vi "Resize and Align.vi"(9 "number of channels":i32, 10 "Refnums for Resizing and Alignment":T4, 11 "State in":T1={"Graph Visible Items"={"Plot Legend"=FALSE, "Scale Legend"=FALSE, "Graph Palette"=FALSE, "Cursor Legend"=FALSE, "X Scrollbar"=FALSE}, "View Table"=FALSE, "Table Visible Items"={"Vertical Scrollbar"=FALSE, "Horizontal Scrollbar"=FALSE, "Row Headers"=FALSE, "Column Headers"=FALSE, "Vertical Lines"=FALSE, "Horizontal Lines"=FALSE}, "Header Font"={"Font Name"="", "Size"=0, "Bold"=FALSE, "Italic"=FALSE, "Underline"=FALSE, "Strikeout"=FALSE, "Color"=0}, "Cell Font"={"Font Name"="", "Size"=0, "Bold"=FALSE, "Italic"=FALSE, "Underline"=FALSE, "Strikeout"=FALSE, "Color"=0}, "Description and Tip..."={"Description"="", "Tip"=""}, "Moveable Splitter Position"=0, "Measurement Cursor Configuration"={"XY"={"enable XY"=FALSE, "Position (X)"=[], "Type"=enum."Absolute", "Y reference"=0.0, "color"=0}, "band"={"enable band"=FALSE, "B1"=0.0, "B2"=0.0, "Fixed bandwidth (B2-B1)"=0.0, "B1 color"=0, "B2 color"=0}, "harmonic"={"enable harmonics"=FALSE, "X reference (1X)"=0.0, "Maximum"=0, "Subset"=enum."All", "1X color"=0, "MX color"=0}, "sideband"={"enable sideband"=FALSE, "X center (C)"=0.0, "Sidebands"=0, "X spacing (s)"=0.0, "Center color"=0, "Sideband color"=0}}, "Cursors"={"List"=[], "Tags"=[]}, "X Increment"=0.0, "X Scale"={"Label Visible"=FALSE, "Label Text"="", "Mapping Mode"=0, "Format String"=""}, "Y Scale"={"Label Visible"=FALSE, "Label Text"="", "Mapping Mode"=0, "Format String"=""}, "Colors"={"background"=16777215, "major grid"=8355711, "minor grid"=12632256, "font"=0}, "desired spectrum view"={"scaling"={"linear/dB"=enum."no change", "dB reference"=0.0, "power/magnitude"=enum."no change", "view"=enum."no change"}, "spectral density"=enum."no change"}, "Plot Color Wheel"=[3381759, 32768, 982784, 4375295, 13827953, 13457919, 16757522, 4343295, 16728758, 12095254], "Plots"=[], "registered user events"=variant, "Lock 1X to Peak"=FALSE} caption="State" {"Y Scale"."Mapping Mode" items=["Linear", "Logarithmic", "dB"]; "X Scale"."Mapping Mode" items=["Linear", "Logarithmic"]}) -> (0 "error out":errorcluster, 3 "State out":T1={"Graph Visible Items"={"Plot Legend"=FALSE, "Scale Legend"=FALSE, "Graph Palette"=FALSE, "Cursor Legend"=FALSE, "X Scrollbar"=FALSE}, "View Table"=FALSE, "Table Visible Items"={"Vertical Scrollbar"=FALSE, "Horizontal Scrollbar"=FALSE, "Row Headers"=FALSE, "Column Headers"=FALSE, "Vertical Lines"=FALSE, "Horizontal Lines"=FALSE}, "Header Font"={"Font Name"="", "Size"=0, "Bold"=FALSE, "Italic"=FALSE, "Underline"=FALSE, "Strikeout"=FALSE, "Color"=0}, "Cell Font"={"Font Name"="", "Size"=0, "Bold"=FALSE, "Italic"=FALSE, "Underline"=FALSE, "Strikeout"=FALSE, "Color"=0}, "Description and Tip..."={"Description"="", "Tip"=""}, "Moveable Splitter Position"=0, "Measurement Cursor Configuration"={"XY"={"enable XY"=FALSE, "Position (X)"=[], "Type"=enum."Absolute", "Y reference"=0.0, "color"=0}, "band"={"enable band"=FALSE, "B1"=0.0, "B2"=0.0, "Fixed bandwidth (B2-B1)"=0.0, "B1 color"=0, "B2 color"=0}, "harmonic"={"enable harmonics"=FALSE, "X reference (1X)"=0.0, "Maximum"=0, "Subset"=enum."All", "1X color"=0, "MX color"=0}, "sideband"={"enable sideband"=FALSE, "X center (C)"=0.0, "Sidebands"=0, "X spacing (s)"=0.0, "Center color"=0, "Sideband color"=0}}, "Cursors"={"List"=[], "Tags"=[]}, "X Increment"=0.0, "X Scale"={"Label Visible"=FALSE, "Label Text"="", "Mapping Mode"=0, "Format String"=""}, "Y Scale"={"Label Visible"=FALSE, "Label Text"="", "Mapping Mode"=0, "Format String"=""}, "Colors"={"background"=16777215, "major grid"=8355711, "minor grid"=12632256, "font"=0}, "desired spectrum view"={"scaling"={"linear/dB"=enum."no change", "dB reference"=0.0, "power/magnitude"=enum."no change", "view"=enum."no change"}, "spectral density"=enum."no change"}, "Plot Color Wheel"=[3381759, 32768, 982784, 4375295, 13827953, 13457919, 16757522, 4343295, 16728758, 12095254], "Plots"=[], "registered user events"=variant, "Lock 1X to Peak"=FALSE} caption="State" {"Y Scale"."Mapping Mode" items=["Linear", "Logarithmic", "dB"]; "X Scale"."Mapping Mode" items=["Linear", "Logarithmic"]})   [LabVIEW 2017, in "Octave with Cursors.xctl"]
doc: "Based on moveable splitter position and pane sizes, resize the graph and table and align table with plot area."
uses:
  <vilib>/addons/_XControls/Octave with Cursors/Octave with Cursors.xctl
  <vilib>/addons/_XControls/Octave with Cursors/Controls/Refnums Typedef.ctl
  <vilib>/addons/Sound and Vibration/svt_Controls/subVIs/Multiplot Octave Graph.ctl
  <vilib>/addons/_XControls/Octave with Cursors/Controls/State.ctl
  <vilib>/Utility/miscctls.llb/LVFontTypeDef.ctl
  <vilib>/addons/_XControls/Octave with Cursors/Controls/Measurement Cursor Configuration.ctl
  <vilib>/Utility/miscctls.llb/LVPositionTypeDef.ctl
  <vilib>/Utility/miscctls.llb/LVRowAndColumnTypeDef.ctl
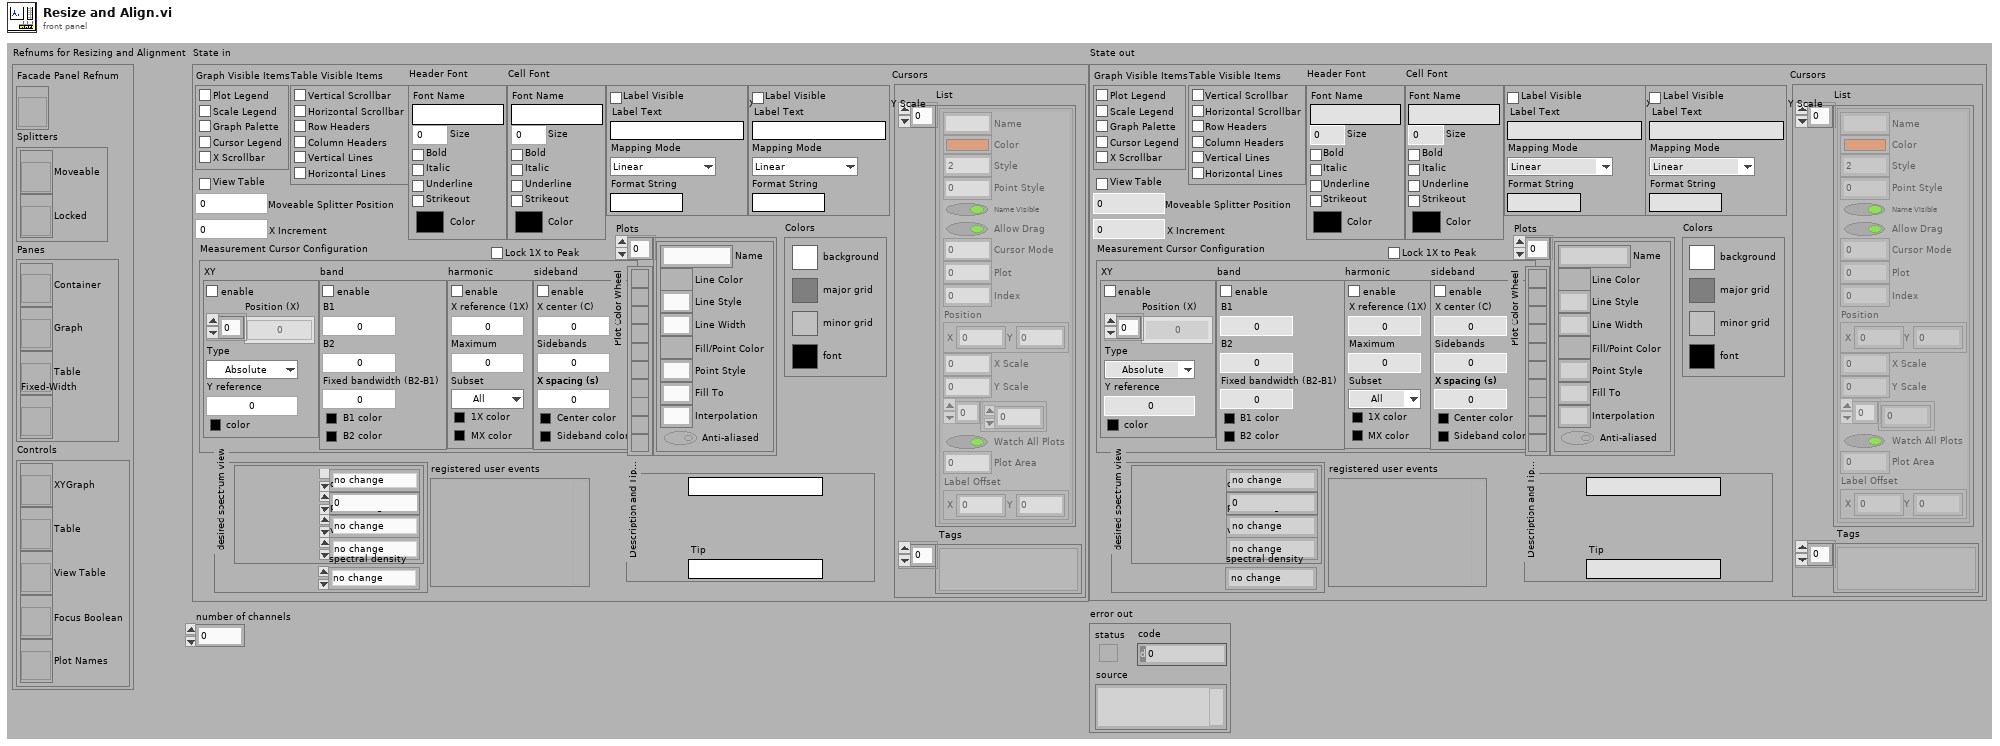
[diagram p1: front panel]
types:
  T1 = typedef "Octave with Cursors.xctl/State.ctl" = cluster{"Graph Visible Items":cluster{"Plot Legend":bool, "Scale Legend":bool, "Graph Palette":bool, "Cursor Legend":bool, "X Scrollbar":bool}, "View Table":bool, "Table Visible Items":cluster{"Vertical Scrollbar":bool, "Horizontal Scrollbar":bool, "Row Headers":bool, "Column Headers":bool, "Vertical Lines":bool, "Horizontal Lines":bool}, "Header Font":T2, "Cell Font":T2, "Description and Tip...":cluster{"Description":string, "Tip":string}, "Moveable Splitter Position":i32, "Measurement Cursor Configuration":T3, "Cursors":cluster{"List":cluster{"Name":string, "Color":u32, "Style":i32, "Point Style":u8, "Name Visible":bool, "Allow Drag":bool, "Cursor Mode":u32, "Plot":i32, "Index":i32, "Position":cluster{"X":dbl, "Y":dbl}, "X Scale":u32, "Y Scale":u32, "Watch Plots":i32[], "Watch All Plots":bool, "Plot Area":i32, "Label Offset":cluster{"X":dbl, "Y":dbl}}[], "Tags":variant[]}, "X Increment":dbl, "X Scale":cluster{"Label Visible":bool, "Label Text":string, "Mapping Mode":u8, "Format String":string}, "Y Scale":cluster{"Label Visible":bool, "Label Text":string, "Mapping Mode":u8, "Format String":string}, "Colors":cluster{"background":u32, "major grid":u32, "minor grid":u32, "font":u32}, "desired spectrum view":cluster{"scaling":cluster{"linear/dB":enum16{"no change", "linear", "dB"}, "dB reference":dbl, "power/magnitude":enum16{"no change", "power", "magnitude"}, "view":enum16{"no change", "rms", "peak", "peak-peak"}}, "spectral density":enum16{"no change", "spectrum", "spectral density"}}, "Plot Color Wheel":u32[], "Plots":cluster{"Name":string, "Line Color":u32, "Line Style":u8, "Line Width":u8, "Fill/Point Color":u32, "Point Style":u8, "Fill To":i16, "Interpolation":u8, "Anti-aliased":bool}[], "registered user events":variant, "Lock 1X to Peak":bool}
  T2 = typedef "LVFontTypeDef.ctl" = cluster{"Font Name":string, "Size":u16, "Bold":bool, "Italic":bool, "Underline":bool, "Strikeout":bool, "Color":u32}
  T3 = typedef "Octave with Cursors.xctl/Measurement Cursor Configuration.ctl" = cluster{"XY":cluster{"enable XY":bool, "Position (X)":dbl[], "Type":enum16{"Absolute", "Relative"}, "Y reference":dbl, "color":u32}, "band":cluster{"enable band":bool, "B1":dbl, "B2":dbl, "Fixed bandwidth (B2-B1)":dbl, "B1 color":u32, "B2 color":u32}, "harmonic":cluster{"enable harmonics":bool, "X reference (1X)":dbl, "Maximum":i32, "Subset":enum16{"All", "Even", "Odd"}, "1X color":u32, "MX color":u32}, "sideband":cluster{"enable sideband":bool, "X center (C)":dbl, "Sidebands":i32, "X spacing (s)":dbl, "Center color":u32, "Sideband color":u32}}
  T4 = typedef "Octave with Cursors.xctl/Refnums Typedef.ctl" = cluster{"Facade Panel Refnum":refnum<vi>, "Splitters":cluster{"Moveable":refnum<vi>, "Locked":refnum<vi>}, "Panes":cluster{"Container":refnum<vi>, "Graph":refnum<vi>, "Table":refnum<vi>, "Fixed-Width":refnum<vi>}, "Controls":cluster{"XYGraph":refnum<vi>, "Table":refnum<vi>, "View Table":refnum<vi>, "Focus Boolean":refnum<vi>, "Plot Names":refnum<vi>}}
  T5 = typedef "LVPositionTypeDef.ctl" = cluster{"Left":i32, "Top":i32}
  T6 = typedef "LVRectTypeDef.ctl" = cluster{"Left":i16, "Top":i16, "Right":i16, "Bottom":i16}
  T7 = typedef "Multiplot Octave Graph.ctl" = cluster{"nominal frequencies [Hz]":dbl[], "band power [dB EU]":dbl[]}[]
  T8 = typedef "LVRowAndColumnTypeDef.ctl" = cluster{"Row":i32, "Column":i32}
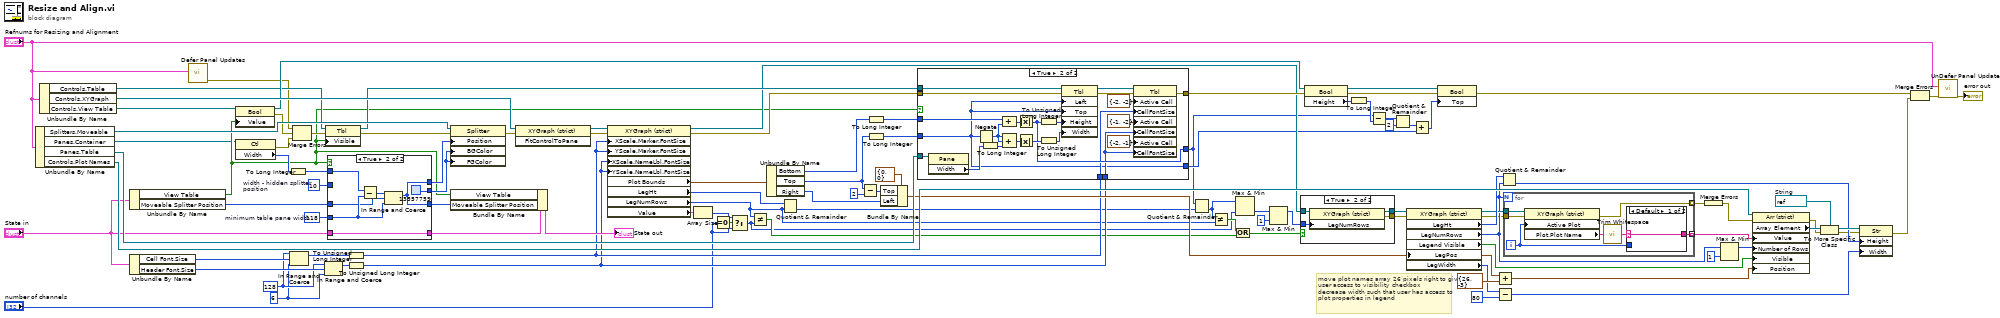
[diagram p0: block diagram]
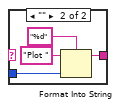
[diagram p3: hidden frame]
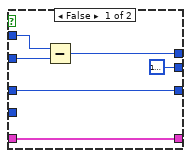
[diagram p4: hidden frame]
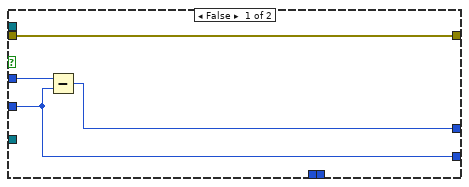
[diagram p5: hidden frame]
diagram:
  w57 = u16 128 ("upper limit")
  w56 = u16 6 ("lower limit")
  w76 = refnum<vi> refnum  # String
  w77 = 118  # minimum table pane width
  w7 = 10  # width - hidden splitter position
  # "move plot names array 26 pixels right to give user access to visibility checkbox\ndecrease width such that user has access to plot properties in legend"
  n1 = Unbundle By Name("Refnums for Resizing and Alignment") -> ("Splitters.Moveable"=w97:refnum<vi>, "Panes.Container"=w5:refnum<vi>, "Panes.Table"=w93:refnum<vi>, "Controls.Plot Names"=w62:refnum<vi>)
  n2 = Unbundle By Name("Refnums for Resizing and Alignment") -> ("Controls.Table"=w17:refnum<vi>, "Controls.XYGraph"=w99:refnum<vi>, "Controls.View Table"=w18:refnum<vi>)
  n3 = Unbundle By Name("State in") -> ("View Table"=w6:bool, "Moveable Splitter Position"=w91:i32)
  n4 = Unbundle By Name("State in") -> ("Cell Font.Size"=w58:u16, "Header Font.Size"=w59:u16)
  n5 = call <vilib>:"Defer Panel Updates.vi"("Refnums for FP Objects"="Refnums for Resizing and Alignment") -> ("error out"=w3:errorcluster)  [unwired: 9 in, 1 out]
  n6 = property class="Bool"(reference=w18, "Value"=w6) -> (reference out=w90:refnum<vi>, error out=w8:errorcluster)  [unwired: 1 in]
  n7 = property class="Ctl"(reference=w5) -> (error out=w98:errorcluster, "Width"=w96:u32)  [unwired: 1 in, 1 out]
  n8 = To Long Integer(number=w96) -> (32bit integer=w79:i32)
  n9 = In Range and Coerce(upper limit=w57, x=w58, lower limit=w56) -> (coerced(x)=w53:u16)  [unwired: 1 out]
  n10 = Merge Errors(w3, w8, w98) -> (w11:errorcluster)
  n11 = In Range and Coerce(upper limit=w57, x=w59, lower limit=w56) -> (coerced(x)=w52:u16)  [unwired: 1 out]
  n12 = property class="Tbl"(reference=w17, error in=w11, "Visible"=w6) -> (reference out=w54:refnum<vi>, error out=w55:errorcluster)
  n13 = case shown="True" w6 {
    tunnel: w79 -> [w106 w114]
    tunnel: [w104 w115] -> w95
    tunnel: [u32 16777216 ("Color Box") u32 13557759 ("Color Box")] -> w94
    tunnel: [w108 w115] -> w78
    tunnel: w91 -> [w108 w110]
    tunnel: w77 -> [_ w113]
    tunnel: "State in" -> [w107 w112]
    tunnel: [w107 w112] -> w10
    tunnel: w7 -> [w105 _]
    frame False {
      n14 = Subtract(x=w106, y=w105) -> (x-y=w104:i32)
    }
    frame True {
      n15 = Subtract(x=w114, y=w113) -> (x-y=w116:i32)
      n16 = In Range and Coerce(upper limit=w116, x=w110, lower limit=w113) -> (coerced(x)=w115:i32)  [unwired: 1 out]
    }
  }
  n17 = To Unsigned Long Integer(number=w53) -> (unsigned 32bit integer=w51:u32)
  n18 = To Unsigned Long Integer(number=w52) -> (unsigned 32bit integer=w50:u32)
  n19 = property class="Splitter"(reference=w97, error in=w55, "Position"=w95, "BGColor"=w94, "FGColor"=w94) -> (error out=w101:errorcluster)  [unwired: 1 out]
  n20 = Bundle By Name(cluster=w10, "View Table"=w6, "Moveable Splitter Position"=w78) -> (→"State out":T1)
  n21 = invoke class="XYGraph (strict)" method="FitControlToPane"(reference=w99, error in=w101) -> (reference out=w103:refnum<vi>, error out=w102:errorcluster)  [unwired: 1 in, 1 out]
  n22 = property class="XYGraph (strict)"(reference=w103, error in=w102, "XScale.Marker.FontSize"=w51, "YScale.Marker.FontSize"=w51, "XScale.NameLbl.FontSize"=w50, "YScale.NameLbl.FontSize"=w50) -> (reference out=w38:refnum<vi>, error out=w100:errorcluster, "Plot Bounds"=w46:T6, "LegHt"=w24:u32, "LegNumRows"=w20:u32, "Value"=w28:T7)
  n23 = Array Size(array=w28) -> (size(s)=w26:i32)
  n24 = Equal To 0?(x="number of channels") -> (x = 0?=w27:bool)
  n25 = Select(t=w26, s=w27, f="number of channels") -> (s? t:f=w13:i32)
  n26 = Not Equal?(x=w20, y=w13) -> (x != y?=w29:bool)
  n27 = Unbundle By Name(w46) -> ("Bottom"=w45:i16, "Top"=w68:i16, "Right"=w69:i16)
  n28 = Quotient & Remainder(x=w24, y=w20) -> (floor(x/y)=w22:u32)  [unwired: 1 out]
  n29 = Subtract(x=w68, y=i16 2) -> (x-y=w67:i16)
  n30 = To Long Integer(number=w45) -> (32bit integer=w80:i32)
  n31 = To Long Integer(number=w68) -> (32bit integer=w49:i32)
  n32 = Bundle By Name(cluster=T5 {"Left"=0, "Top"=0} ("Legend:Position"), "Top"=w67, "Left"=w69) -> (w60:T5)
  n33 = case shown="True" w6 {
    tunnel: w54 -> [_ w142]
    tunnel: w49 -> [w117 w121]
    tunnel: w80 -> [w119 w141]
    tunnel: w93 -> [_ w139]
    tunnel: w100 -> [w120 w136]
    tunnel: [w120 w122] -> w87
    tunnel: [w118 w128] -> w21
    tunnel: w51 -> [_ w126]
    tunnel: w50 -> [_ w123]
    tunnel: [w117 w121] -> w23
    frame False {
      n34 = Subtract(x=w119, y=w117) -> (x-y=w118:i32)
    }
    frame True {
      n35 = property class="Pane"(reference=w139) -> ("Width"=w138:u32)  [unwired: 1 in, 2 out]
      n36 = Negate(x=w121) -> (-x=w133:i32)
      n37 = To Long Integer(number=w138) -> (32bit integer=w134:i32)
      n38 = Compound Arithmetic op=ADD(w141, w133) -> (w140:i32)
      n39 = Compound Arithmetic op=ADD(w133, w133, w134) -> (w137:i32)
      n40 = Absolute Value(x=w140) -> (abs(x)=w128:i32)
      n41 = Absolute Value(x=w137) -> (abs(x)=w131:i32)
      n42 = To Unsigned Long Integer(number=w128) -> (unsigned 32bit integer=w135:u32)
      n43 = To Unsigned Long Integer(number=w131) -> (unsigned 32bit integer=w132:u32)
      n44 = property class="Tbl"(reference=w142, error in=w136, "Left"=w121, "Top"=w121, "Height"=w135, "Width"=w132) -> (reference out=w130:refnum<vi>, error out=w129:errorcluster)
      n45 = property class="Tbl"(reference=w130, error in=w129, "Active Cell"=T8 {"Row"=-2, "Column"=-2} ("Active Cell:Active Cell"), "CellFontSize"=w126, "Active Cell"=T8 {"Row"=-1, "Column"=-2} ("Active Cell:Active Cell"), "CellFontSize"=w123, "Active Cell"=T8 {"Row"=-2, "Column"=-1} ("Active Cell:Active Cell"), "CellFontSize"=w123) -> (error out=w122:errorcluster)  [unwired: 1 out]
    }
  }
  n46 = Quotient & Remainder(x=w21, y=w22) -> (floor(x/y)=w14:u32)  [unwired: 1 out]
  n47 = Not Equal?(x=w14, y=w20) -> (x != y?=w19:bool)
  n48 = Or(x=w19, y=w29) -> (x .or. y?=w30:bool)
  n49 = Max & Min(x=w14, y=w13) -> (min(x,y)=w15:u32)  [unwired: 1 out]
  n50 = Max & Min(x=w15, y=u32 1 ("lower limit")) -> (max(x,y)=w12:u32)  [unwired: 1 out]
  n51 = case shown="True" w30 {
    tunnel: w38 -> [w143 w147]
    tunnel: [w143 w146] -> w37
    tunnel: w12 -> [_ w145]
    tunnel: [_ w144] -> w36
    frame False {
    }
    frame True {
      n52 = property on="Property Node" class="XYGraph (strict)"(reference=w147, "LegNumRows"=w145) -> (reference out=w146:refnum<vi>, error out=w144:errorcluster)  [unwired: 1 in]
    }
  }
  n53 = property class="Bool"(reference=w90, error in=w87) -> (reference out=w89:refnum<vi>, error out=w86:errorcluster, "Height"=w88:u32)
  n54 = To Long Integer(number=w88) -> (32bit integer=w85:i32)
  n55 = Subtract(x=w21, y=w85) -> (x-y=w84:i32)
  n56 = Quotient & Remainder(x=w84, y=2) -> (floor(x/y)=w82:i32)  [unwired: 1 out]
  n57 = property on="Property Node" class="XYGraph (strict)"(reference=w37, error in=w36, "LegPos"=w60) -> (reference out=w43:refnum<vi>, error out=w35:errorcluster, "LegHt"=w47:u32, "LegNumRows"=w39:u32, "Legend Visible"=w48:bool, "LegWidth"=w61:u32)
  n58 = Add(x=w82, y=w23) -> (x+y=w81:i32)
  n59 = property class="Bool"(reference=w89, error in=w86, "Top"=w81) -> (error out=w41:errorcluster)  [unwired: 1 out]
  n60 = Add(x=w60, y=T5 {"Left"=26, "Top"=-3}) -> (x+y=w72:T5)
  n61 = Subtract(x=w61, y=u32 80) -> (x-y=w63:u32)
  n62 = Quotient & Remainder(x=w47, y=w39) -> (floor(x/y)=w66:u32)  [unwired: 1 out]
  n63 = for {
    N: w39 -> [_]
    tunnel: [w154] -> w64 mode=indexing
    tunnel: w43 -> [w153]
    tunnel: w35 -> [w149]
    tunnel: [w148] -> w34 mode=indexing
    i -> [w150]
    n64 = property on="Property Node" class="XYGraph (strict)"(reference=w153, error in=w149, "Active Plot"=w150) -> (error out=w148:errorcluster, "Plot.Plot Name"=w152:string)  [unwired: 1 out]
    n65 = call <vilib>:"Trim Whitespace.vi"("string"=w152) -> ("trimmed string"=w151:string)  [unwired: 1 in]
    n66 = case shown="Default" w151 {
      selector: w151 -> [w155 _]
      tunnel: w150 -> [_ w159]
      tunnel: [w155 w156] -> w154
      frame Default {
      }
      frame "" {
        n67 = Format Into String(format string="%d", initial string="Plot ", w159) -> (resulting string=w156:string)  [unwired: 1 in, 1 out]
      }
    }
  }
  n68 = Merge Errors(w34) -> (w33:errorcluster)
  n69 = Max & Min(x=w39, y=u32 1 ("lower limit")) -> (max(x,y)=w42:u32)  [unwired: 1 out]
  n70 = property on="Property Node" class="Arr (strict)"(reference=w62, error in=w33, "Value"=w64, "Number of Rows"=w42, "Visible"=w48, "Position"=w72) -> (error out=w32:errorcluster, "Array Element"=w65:refnum<vi>)  [unwired: 1 out]
  n71 = To More Specific Class(target class=w76, reference=w65, error in=w32) -> (specific class reference=w75:refnum<vi>, error out=w31:errorcluster)
  n72 = property class="Str"(reference=w75, error in=w31, "Height"=w66, "Width"=w63) -> (error out=w40:errorcluster)  [unwired: 1 out]
  n73 = Merge Errors(w41, w40) -> (w4:errorcluster)
  n74 = call <vilib>:"UnDefer Panel Updates.vi"("error in (no error)"=w4, "Refnums for FP Objects"="Refnums for Resizing and Alignment") -> ("error out"=→"error out":errorcluster)  [unwired: 8 in, 1 out]
